vi "String EQ.vi"(11 "Data In":string) -> (3 "Data Out":string)   [LabVIEW 2016]
uses:
  Core/Assert API Components/Failure Actions.ctl
  Core/Assert API Components/Assert API Components.lvlib
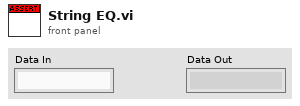
[diagram p1: front panel]
types:
  T1 = typedef "Assert API Components.lvlib/Failure Actions.ctl" = enum16{"None", "Log To File", "Pause Execution", "Abort Execution"}
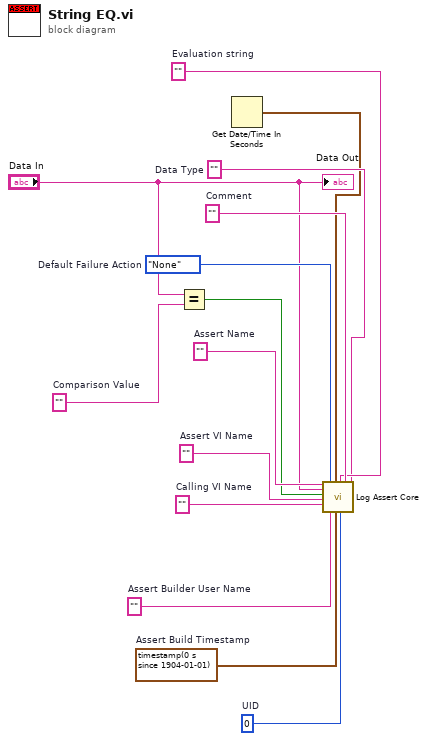
[diagram p0: block diagram]
diagram:
  w1 = 0  # UID
  w3 = ""  # Assert VI Name
  w4 = ""  # Calling VI Name
  w5 = timestamp(0 s since 1904-01-01)  # Assert Build Timestamp
  w6 = ""  # Assert Builder User Name
  w7 = ""  # Data Type
  w11 = ""  # Comment
  w8 = ""  # Evaluation string
  w13 = Failure_Actions."None"  # Default Failure Action
  w14 = ""  # Assert Name
  w12 = ""  # Comparison Value
  n1 = Equal?(x="Data In", y=w12) -> (x = y?=w9:bool)
  n2 = Get Date/Time In Seconds() -> (seconds since 1Jan1904=w2:timestamp)
  n3 = call "Log Assert Core.vi"("Assert Name"=w14, "Data Value"="Data In", "Status"=w9, "Assert VI Name"=w3, "Calling VI Name"=w4, "Failure Action"=w13, "Assert Builder User Name"=w6, "Last Update"=w2, "Assert Build Timestamp"=w5, "Evaluation String"=w8, "Assert VI UID"=w1, "Comment"=w11, "Data Type"=w7) -> ()  [unwired: 7 in]
  "Data Out" <- "Data In"
